vi "overlay LED colors.vi"(10 "BASE ARRAY":u32[](array[colorbox]), 11 "OVERLAY":u32[](array[colorbox])) -> (3 "BLENDED ARRAY":u32[](array[colorbox]))   [LabVIEW 2023]
panel:
  out "max color value":dbl
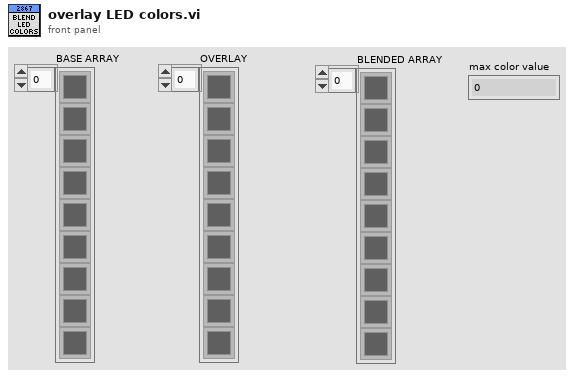
[diagram p1: front panel]
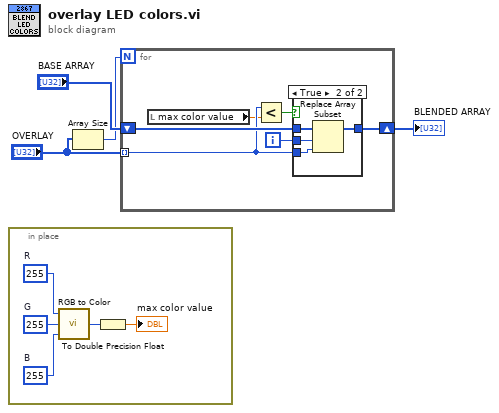
[diagram p0: block diagram]
diagram:
  n1 = in-place {
    w8 = u8 255  # G
    w9 = u8 255  # B
    w7 = u8 255  # R
    n2 = call <vilib>:"RGB to Color.vi"("B"=w9, "G"=w8, "R"=w7) -> ("Color"=w6:u32)
    n3 = To Double Precision Float(number=w6) -> (double precision float=→"max color value":dbl)
  }
  n4 = Array Size(array="OVERLAY") -> (size(s)=w2:i32)
  n5 = for {
    N: w2 -> [_]
    tunnel: "OVERLAY" -> [w12] mode=indexing
    shift-right: [w14] -> w4
    shift-left: "BASE ARRAY" -> [w15]
    i -> [w13]
    n6 = local read "max color value"() -> (w10:dbl)
    n7 = Less?(x=w12, y=w10) -> (x < y?=w11:bool)
    n8 = case shown="True" w11 {
      tunnel: w15 -> [w16 w20]
      tunnel: [w16 w19] -> w14
      tunnel: w13 -> [_ w18]
      tunnel: w12 -> [_ w17]
      frame False {
      }
      frame True {
        n9 = Replace Array Subset(array=w20, new element=w17, index=w18) -> (w19:u32[])
      }
    }
  }
  "BLENDED ARRAY" <- w4
